vi "Add Sub Object.vi"(8 "error in":errorcluster, 10 "Sub Object":refnum<class "Sub Object.lvclass">, 11 "Obj Entry in":refnum<class "Object Entry.lvclass">) -> (0 "error out":errorcluster, 3 "Obj Entry out":refnum<class "Object Entry.lvclass">)   [LabVIEW 2020, in "CANopen.lvlib" / "Object Entry.lvclass"]
doc: "Adds an entry with the specified key and value into the Ordered Dictionary collection with the lowest available index."
uses:
  Object Entry.lvclass
  Sub Object/Sub Object.lvclass
  Object Entry.lvclass/Object Entry.ctl
  Sub Objects Dictionary/Sub Objects Dictionary.lvclass
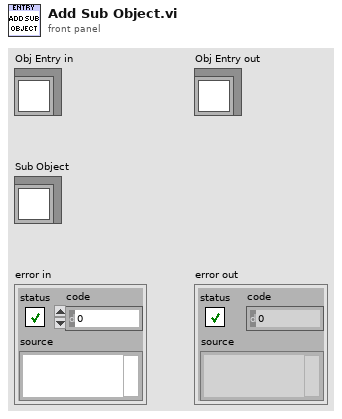
[diagram p1: front panel]
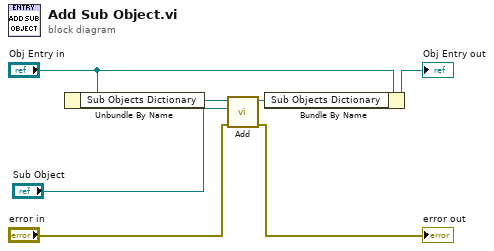
[diagram p0: block diagram]
diagram:
  n1 = Unbundle By Name("Obj Entry in") -> ("Sub Objects Dictionary"=w6:refnum<class "Sub Objects Dictionary.lvclass">)
  n2 = call "Add.vi"("error in"="error in", "Sub Object"="Sub Object", "Sub Objects Dictionary in"=w6) -> ("error out"=→"error out":errorcluster, "Sub Objects Dictionary out"=w1:refnum<class "Sub Objects Dictionary.lvclass">)  [unwired: 7 in]
  n3 = Bundle By Name(cluster="Obj Entry in", "Sub Objects Dictionary"=w1) -> (→"Obj Entry out":refnum<class "Object Entry.lvclass">)
